vi "NavX Global Data.vi"() -> ()   [LabVIEW 2015]
uses:
  navX-MXP Library/COMMON/TypeDefs/Data TypeDefs/navX YPRH Data.ctl
  navX-MXP Library/navX-MXP IMU.lvlib
panel:
  out "YPRH":T1
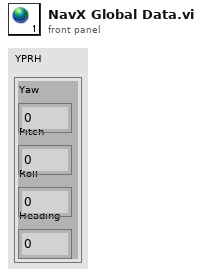
[diagram p1: front panel]
types:
  T1 = typedef "navX-MXP IMU.lvlib/navX YPRH Data.ctl" = cluster{"Yaw":dbl, "Pitch":dbl, "Roll":dbl, "Heading":dbl}
diagram:
